vi "Timer.vi"(8 "error in (no error)":errorcluster, 9 "Message Queue":refnum<queue>, 10 "Event Registration Refnum":refnum<event-registration>, 11 "Timer Handler":T1) -> (0 "error out":errorcluster, 3 "dup Timer Handler":T1)   [LabVIEW 2024]
doc: "Functions as the main timer loop."
uses:
  Shared/Message Queue/Message Cluster.ctl
  Timer Handler.ctl
  Timer Parameter.ctl
  Shared/Message Queue.lvlib
panel:
  out "Timer Interval (hours)":u32
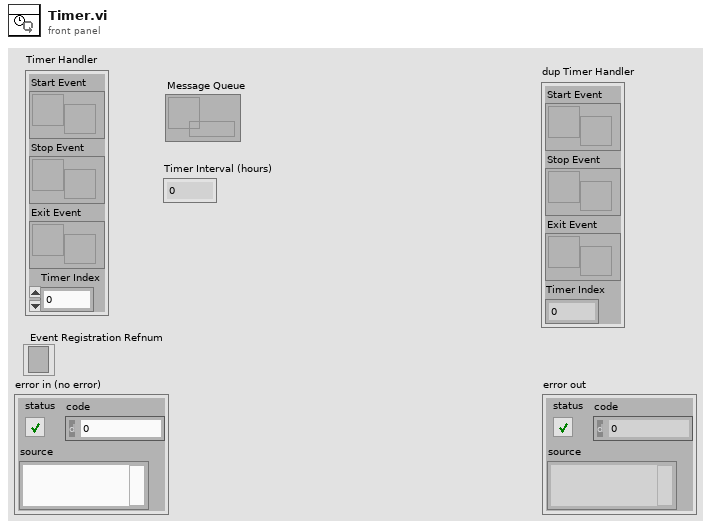
[diagram p1: front panel]
types:
  T1 = typedef "Timer Handler.ctl" = cluster{"Start Event":refnum<user-event>, "Stop Event":refnum<user-event>, "Exit Event":refnum<user-event>, "Timer Index":u32}
  T2 = typedef "Timer Parameter.ctl" = cluster{"Index":u32, "Value":variant}
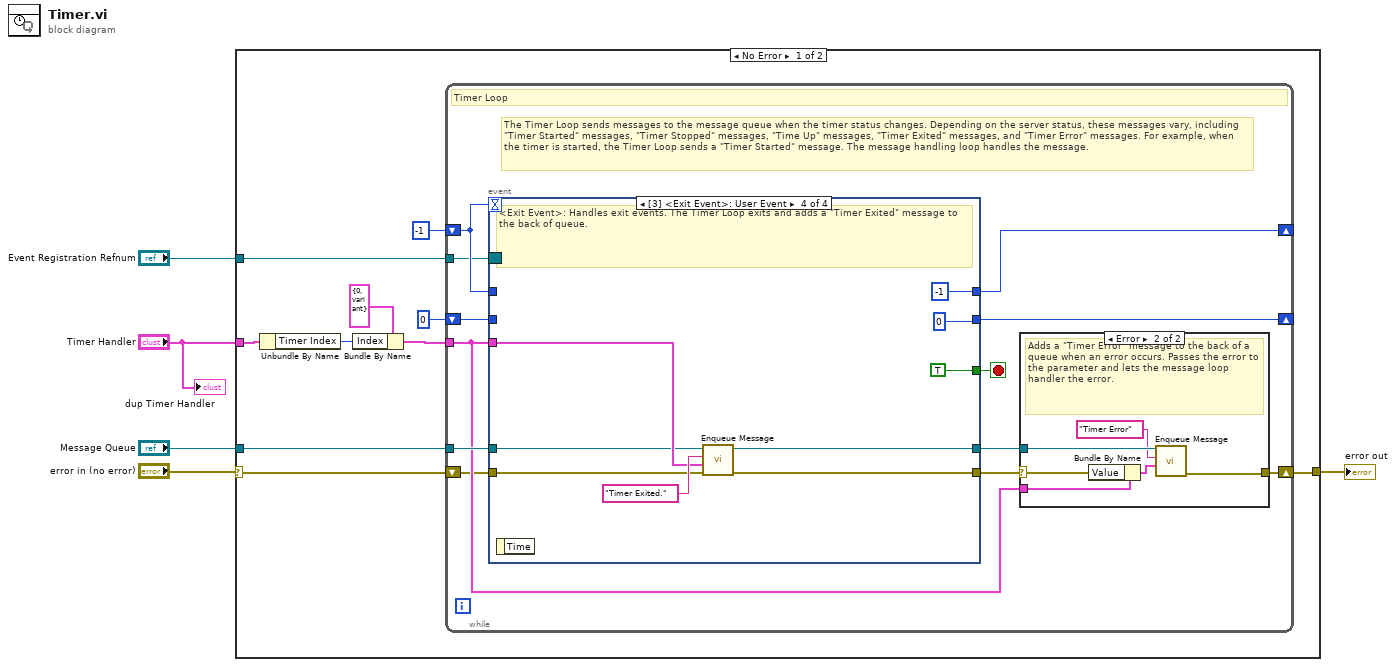
[diagram p0: block diagram]
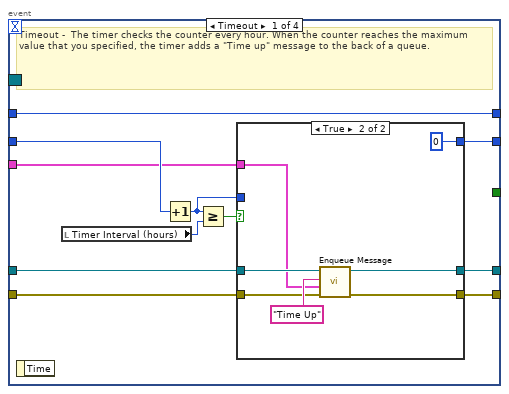
[diagram p3: hidden frame]
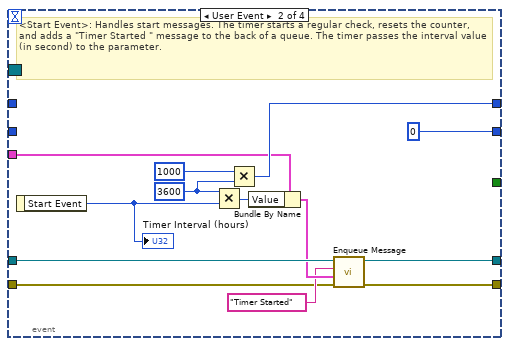
[diagram p5: hidden frame]
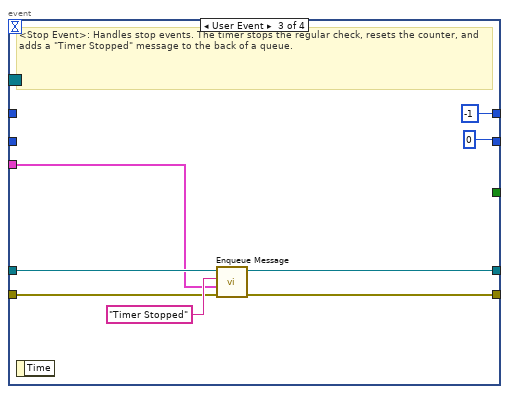
[diagram p6: hidden frame]
diagram:
  n1 = case shown="No Error" "error in (no error)" {
    selector: "error in (no error)" -> [w6 w86]
    tunnel: [w11 w86] -> w4
    tunnel: "Timer Handler" -> [w10 _]
    tunnel: "Event Registration Refnum" -> [w8 _]
    tunnel: "Message Queue" -> [w7 _]
    frame No Error {
      n2 = Unbundle By Name(w10) -> ("Timer Index"=w13:u32)
      n3 = Bundle By Name(cluster=T2 {"Index"=0, "Value"=variant} ("Alarm Parameter"), "Index"=w13) -> (w12:T2)
      n4 = while {
        tunnel: w7 -> [w26]
        shift-right: [w25] -> _
        shift-left: 0 ("Delay Time (hours)") -> [w24]
        shift-right: [w23] -> _
        shift-left: -1 -> [w22]
        tunnel: w8 -> [w21]
        tunnel: w12 -> [w17]
        shift-right: [w19] -> w11
        shift-left: w6 -> [w16]
        stop <- w27 stop-if-true
        # "The Timer Loop sends messages to the message queue when the timer status changes. Depending on the server status, these messages vary, including \"Timer Started\" messages, \"Timer Stopped\" messages, \"Time Up\" messages, \"Timer Exited\" messages, and \"Timer Error\" messages. For example, when the timer is started, the Timer Loop sends a \"Timer Started\" message. The message handling loop handles the message."
        # "Timer Loop"
        n5 = event shown="[3] <Exit Event>: User Event" {
          selector: w21 -> [_ _ _ _]
          dyn-events: _ -> [_ _ _ _]
          timeout: w22 -> [_ _ _ _]
          tunnel: [_ _ _ TRUE ("Stop?")] -> w27
          tunnel: w26 -> [w45 w64 w73 w80]
          tunnel: [w43 0 ("Delay Time (s)") 0 ("Delay Time (hours)") 0 ("Delay Time (hours)")] -> w25
          tunnel: w24 -> [w44 _ _ _]
          tunnel: [w40 w68 -1 ("Delay Time (s)") -1] -> w23
          tunnel: w22 -> [w40 _ _ _]
          tunnel: w17 -> [w38 w60 w72 w81]
          tunnel: [w39 w59 w71 w79] -> w20
          tunnel: [w36 w57 w70 w78] -> w18
          tunnel: w16 -> [w35 w56 w69 w77]
          event Timeout {
            # "Timeout -  The timer checks the counter every hour. When the counter reaches the maximum value that you specified, the timer adds a \"Time up\" message to the back of a queue."
            n6 = event-data() -> ()  [unwired: 1 in, 1 out]
            n7 = local read "Timer Interval (hours)"() -> (w37:u32)
            n8 = Increment(x=w44) -> (x+1=w42:i32)
            n9 = Greater Or Equal?(x=w42, y=w37) -> (x >= y?=w41:bool)
            n10 = case shown="True" w41 {
              tunnel: [w48 0 ("Delay Time (hours)")] -> w43
              tunnel: w42 -> [w48 _]
              tunnel: w45 -> [w47 w54]
              tunnel: [w46 w52] -> w39
              tunnel: w38 -> [_ w51]
              tunnel: [w47 w50] -> w36
              tunnel: w35 -> [w46 w49]
              frame False {
              }
              frame True {
                n11 = call "Enqueue Message.vi"("error in (no error)"=w49, "Message Data"=w51, "Message"="Time Up", "Message Queue"=w54) -> ("error out"=w52:errorcluster, "dup Message Queue"=w50:refnum<queue>)  [unwired: 6 in]
              }
            }
          }
          event User Event {
            w67 = 3600 ("Delay Time (s)")
            # "<Start Event>: Handles start messages. The timer starts a regular check, resets the counter, and adds a \"Timer Started \" message to the back of a queue. The timer passes the interval value (in second) to the parameter."
            n12 = event-data() -> ("Start Event"=w58:u32)  [unwired: 1 in]
            "Timer Interval (hours)" <- w58
            n13 = Multiply(x=w67, y=w58) -> (x*y=w63:u32)
            n14 = Multiply(x=1000, y=w67) -> (x*y=w68:i32)
            n15 = Bundle By Name(cluster=w60, "Value"=w63) -> (w62:T2)
            n16 = call "Enqueue Message.vi"("error in (no error)"=w56, "Message Data"=w62, "Message"="Timer Started", "Message Queue"=w64) -> ("error out"=w59:errorcluster, "dup Message Queue"=w57:refnum<queue>)  [unwired: 6 in]
          }
          event User Event {
            # "<Stop Event>: Handles stop events. The timer stops the regular check, resets the counter, and adds a \"Timer Stopped\" message to the back of a queue."
            n17 = event-data() -> ()  [unwired: 1 in, 1 out]
            n18 = call "Enqueue Message.vi"("error in (no error)"=w69, "Message Data"=w72, "Message"="Timer Stopped", "Message Queue"=w73) -> ("error out"=w71:errorcluster, "dup Message Queue"=w70:refnum<queue>)  [unwired: 6 in]
          }
          event User Event {
            # "<Exit Event>: Handles exit events. The Timer Loop exits and adds a \"Timer Exited\" message to the back of queue."
            n19 = event-data() -> ()  [unwired: 1 in, 1 out]
            n20 = call "Enqueue Message.vi"("error in (no error)"=w77, "Message Data"=w81, "Message"="Timer Exited.", "Message Queue"=w80) -> ("error out"=w79:errorcluster, "dup Message Queue"=w78:refnum<queue>)  [unwired: 6 in]
          }
        }
        n21 = case shown="Error" w20 {
          selector: w20 -> [w28 w31]
          tunnel: [w28 w32] -> w19
          tunnel: w18 -> [_ w34]
          tunnel: w17 -> [_ w30]
          frame No Error {
            # "No error case."
          }
          frame Error {
            # "Adds a \"Timer Error\" message to the back of a queue when an error occurs. Passes the error to the parameter and lets the message loop handler the error."
            n22 = Bundle By Name(cluster=w30, "Value"=w31) -> (w29:T2)
            n23 = call "Enqueue Message.vi"("Message Data"=w29, "Message"="Timer Error", "Message Queue"=w34) -> ("error out"=w32:errorcluster)  [unwired: 7 in, 1 out]
          }
        }
      }
    }
    frame Error {
    }
  }
  "error out" <- w4
  "dup Timer Handler" <- "Timer Handler"
